vi "BLM Read Position.vi"(4 "error in (no error)":errorcluster, 5 "Steps/rot":dbl=8000.0, 6 "Motor Address":string="0", 7 "Port Address":refnum<visa-resource-name>) -> (0 "error out":errorcluster, 1 "Response":dbl format="%.4f", 2 "Delta Time":u32, 3 "Port Address Out":refnum<visa-resource-name>)   [LabVIEW 2019]
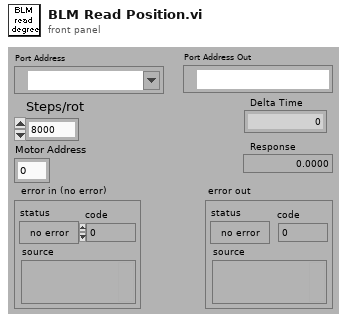
[diagram p1: front panel]
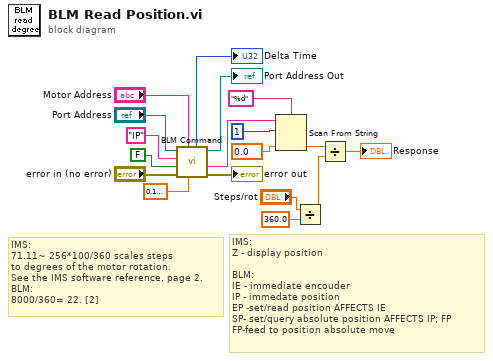
[diagram p0: block diagram]
diagram:
  # "IMS:\nZ - display position\n\nBLM:\nIE - immediate encouder\nIP - immedate position \nEP -set/read position AFFECTS IE\nSP- set/query absolute position AFFECTS IP; FP\nFP-feed to position absolute move"
  # "IMS:\n71.11~ 256*100/360 scales steps\nto degrees of the motor rotation.\nSee the IMS software reference, page 2.\nBLM:\n8000/360= 22. [2]"
  n1 = call "BLM Command.vi"("Timeout Limit"=sgl 0.1, "Motor Address"="Motor Address", "error in (no error)"="error in (no error)", "Read Echo?"=FALSE, "Command"="IP", "Port Address"="Port Address") -> ("error out"=→"error out":errorcluster, "Response"=w12:string, "Port Address Out"=→"Port Address Out":refnum<visa-resource-name>, "Delta Time"=→"Delta Time":u32)  [unwired: 1 out]
  n2 = Scan From String(format string="%d", input string=w12, initial scan location=u32 1, default 1=0.0 ("default value 1")) -> (output 1=w14:dbl)  [unwired: 1 in, 3 out]
  n3 = Divide(x="Steps/rot", y=360.0) -> (x/y=w7:dbl)
  n4 = Divide(x=w14, y=w7) -> (x/y=→"Response":dbl)
